vi "PUREFLDdll.vi"(8 "error in (no error)":errorcluster, 11 "icomp":i32) -> (0 "error out":errorcluster, 3 "icomp out":i32)   [LabVIEW 2016]
doc: "subroutine PUREFLD (icomp)\n\nChange the standard mixture setup so that the properties of one fluid\ncan be calculated as if SETUP had been called for a pure fluid.\n\nCalling this routine will disable all mixture calculations.\nTo reset the mixture setup, call this routine with icomp=0.\n\nINPUTS:\nicomp--fluid number in a mixture to use as a pure fluid"
uses:
  REFPROP.DLL
panel:
  # "REFPROP-PUREFLDdll.vi"
  # "void  PUREFLDdll(int32_t *icomp)"
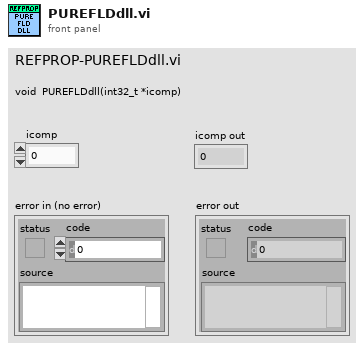
[diagram p1: front panel]
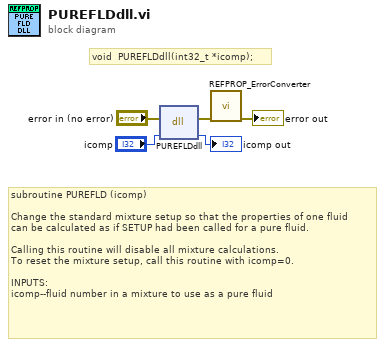
[diagram p0: block diagram]
diagram:
  # "void  PUREFLDdll(int32_t *icomp);"
  # "subroutine PUREFLD (icomp)\n\nChange the standard mixture setup so that the properties of one fluid\ncan be calculated as if SETUP had been called for a pure fluid.\n\nCalling this routine will disable all mixture calculations.\nTo reset the mixture setup, call this routine with icomp=0.\n\nINPUTS:\nicomp--fluid number in a mixture to use as a pure fluid"
  n1 = dll-call lib="S:/009 - Testing/02 - Performance Testing/REFPROP/REFPROP.*" fn="PUREFLDdll"(error in="error in (no error)", "icomp"="icomp") -> (error out=w3:errorcluster, "icomp"=→"icomp out":i32)  [unwired: 3 in, 1 out]
  n2 = call "REFPROP_ErrorConverter.vi"("error in (no error)"=w3) -> ("error out"=→"error out":errorcluster)  [unwired: 10 in]
